vi "Set Do Delay.vi"(10 "Do Delay":i32=1000 format="%d ms", 11 "CAN Task in":refnum<class "CANopen Task Actor.lvclass">) -> (3 "CAN Task out":refnum<class "CANopen Task Actor.lvclass">)   [LabVIEW 2024, in "CANopen Task Actor.lvlib" / "CANopen Task Actor.lvclass"]
uses:
  CANopen Task Actor.lvclass
  CANopen Task Actor.lvclass/CANopen Task Actor.ctl
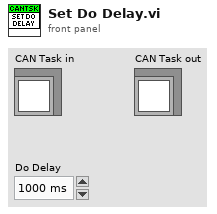
[diagram p1: front panel]
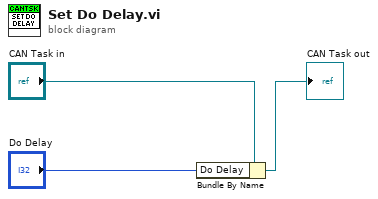
[diagram p0: block diagram]
diagram:
  n1 = Bundle By Name(cluster="CAN Task in", "Do Delay"="Do Delay") -> (→"CAN Task out":refnum<class "CANopen Task Actor.lvclass">)
